vi "Write Modulation timed_.vi"(8 "error in (no error)":errorcluster, 10 "Modulation timed?":bool, 11 "HC-Main in":refnum<class "HC-Main.lvclass">) -> (0 "error out":errorcluster, 3 "HC-Main out":refnum<class "HC-Main.lvclass">)   [LabVIEW 2013, in "HardwareCharacterization.lvlib" / "HC-Main.lvclass"]
uses:
  HC-Main.lvclass
  HC-Main.lvclass/HC-Main.ctl
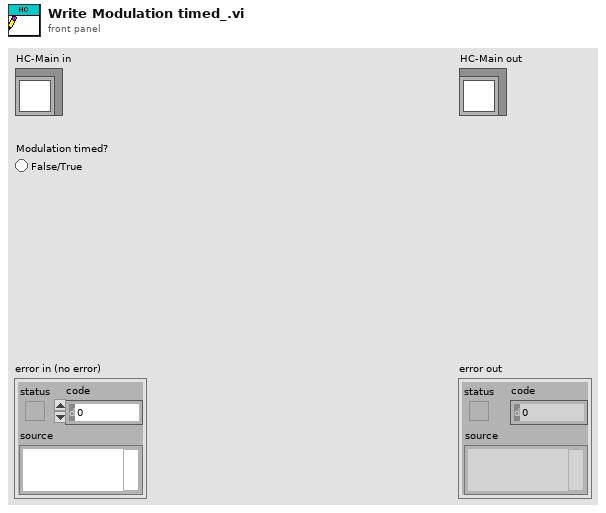
[diagram p1: front panel]
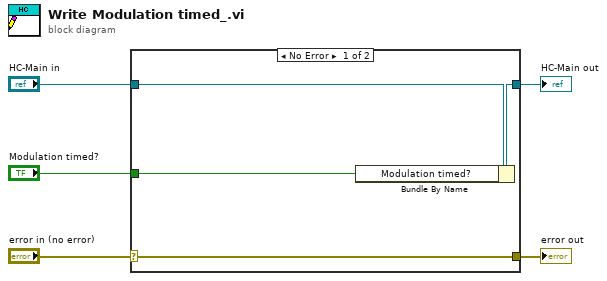
[diagram p0: block diagram]
diagram:
  n1 = case shown="No Error" "error in (no error)" {
    selector: "error in (no error)" -> [w9 w10]
    tunnel: [w9 w10] -> w4
    tunnel: [w7 w11] -> w2
    tunnel: "HC-Main in" -> [w8 w11]
    tunnel: "Modulation timed?" -> [w6 _]
    frame No Error {
      n2 = Bundle By Name(cluster=w8, "Modulation timed?"=w6) -> (w7:refnum<class "HC-Main.lvclass">)
    }
    frame Error {
    }
  }
  "error out" <- w4
  "HC-Main out" <- w2
